vi "Get spec value.vi"(8 "error in (no error)":errorcluster, 10 "Command string":string="P0=", 11 "VISA resource name":refnum<visa-resource-name>) -> (0 "error out":errorcluster, 1 "Value string":string, 2 "Value":dbl, 3 "VISA resource name out":refnum<visa-resource-name>)   [LabVIEW 2020, in "Datron D4xxx.lvlib"]
doc: "This VI sends read-out command (P, U, X or some of V) and returns converted number if value is displayable."
uses:
  Datron D4xxx.lvlib
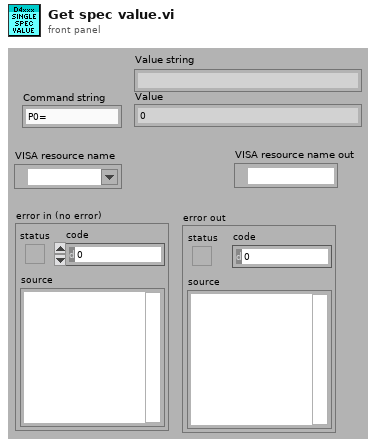
[diagram p1: front panel]
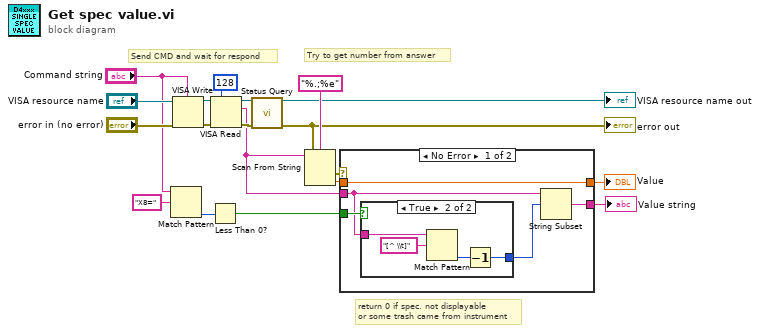
[diagram p0: block diagram]
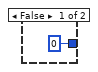
[diagram p2: hidden frame]
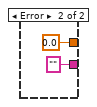
[diagram p3: hidden frame]
diagram:
  # "Try to get number from answer"
  # "return 0 if spec. not displayable\nor some trash came from instrument"
  # "Send CMD and wait for respond"
  n1 = Match Pattern(string="Command string", regular expression="X8=") -> (offset past match=w2:i32)  [unwired: 1 in, 3 out]
  n2 = VISA Write(VISA resource name="VISA resource name", write buffer="Command string", error in (no error)="error in (no error)") -> (VISA resource name out=w16:refnum<visa-resource-name>, error out=w17:errorcluster)  [unwired: 1 out]
  n3 = Less Than 0?(x=w2) -> (x < 0?=w1:bool)
  n4 = VISA Read(VISA resource name=w16, byte count=u32 128, error in (no error)=w17) -> (VISA resource name out=w15:refnum<visa-resource-name>, read buffer=w5:string, error out=w14:errorcluster)  [unwired: 1 out]
  n5 = call "Status Query.vi"("VISA resource name"=w15, "error in (no error)"=w14) -> ("VISA resource name out"=→"VISA resource name out":refnum<visa-resource-name>, "error out"=w10:errorcluster)  [unwired: 5 in, 7 out]
  "error out" <- w10
  n6 = Scan From String(format string="%.;%e", input string=w5, error in=w10) -> (error out=w8:errorcluster, output 1=w6:dbl)  [unwired: 2 in, 2 out]
  n7 = case shown="No Error" w8 {
    tunnel: [w24 0.0] -> w13
    tunnel: w6 -> [w24 _]
    tunnel: w5 -> [w21 _]
    tunnel: [w23 "" ("read buffer")] -> w7
    tunnel: w1 -> [w22 _]
    frame No Error {
      n8 = case shown="True" w22 {
        tunnel: w21 -> [_ w29]
        tunnel: [0 ("offset past match") w26] -> w20
        frame False {
        }
        frame True {
          n9 = Match Pattern(string=w29, regular expression="[^ \\t]") -> (offset past match=w27:i32)  [unwired: 1 in, 3 out]
          n10 = Decrement(x=w27) -> (x-1=w26:i32)
        }
      }
      n11 = String Subset(string=w21, offset (0)=w20) -> (substring=w23:string)  [unwired: 1 in]
    }
    frame Error {
    }
  }
  "Value" <- w13
  "Value string" <- w7
